vi "Transfer_FLSH_Format.vi"(11 "FLSH Outputs":T1={"t"=0.0, "p"=0.0, "D"=0.0, "Dl"=0.0, "Dv"=0.0, "x"=[0.0, 0.0, 0.0, 0.0, 0.0, 0.0, 0.0, 0.0, 0.0, 0.0, 0.0, 0.0, 0.0, 0.0, 0.0, 0.0, 0.0, 0.0, 0.0, 0.0], "y"=[0.0, 0.0, 0.0, 0.0, 0.0, 0.0, 0.0, 0.0, 0.0, 0.0, 0.0, 0.0, 0.0, 0.0, 0.0, 0.0, 0.0, 0.0, 0.0, 0.0], "q"=0.0, "e"=0.0, "h"=0.0, "s"=0.0, "Cv"=0.0, "Cp"=0.0, "w"=0.0, "ierr"=0, "herr"="", "herr_Length"=0}) -> (3 "Array out":dbl[](array[numeric]))   [LabVIEW 2016]
doc: "Converts output clusters from all FLSH functions to an array of data"
uses:
  Ctl/FLSH_Outputs.ctl
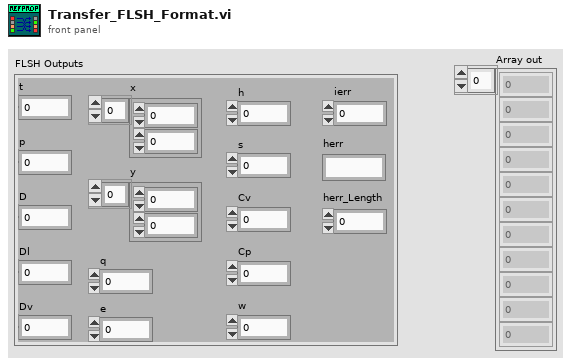
[diagram p1: front panel]
types:
  T1 = typedef "FLSH_Outputs.ctl" = cluster{"t":dbl, "p":dbl, "D":dbl, "Dl":dbl, "Dv":dbl, "x":dbl[], "y":dbl[], "q":dbl, "e":dbl, "h":dbl, "s":dbl, "Cv":dbl, "Cp":dbl, "w":dbl, "ierr":i32, "herr":string, "herr_Length":i32}
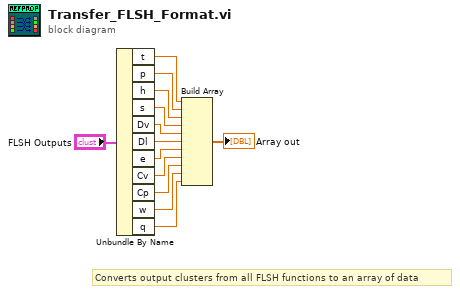
[diagram p0: block diagram]
diagram:
  # "Converts output clusters from all FLSH functions to an array of data"
  n1 = Unbundle By Name("FLSH Outputs") -> ("t"=w11:dbl, "p"=w10:dbl, "h"=w9:dbl, "s"=w8:dbl, "Dv"=w7:dbl, "Dl"=w6:dbl, "e"=w5:dbl, "Cv"=w4:dbl, "Cp"=w3:dbl, "w"=w2:dbl, "q"=w1:dbl)
  n2 = Build Array(w11, w10, w9, w8, w7, w6, w5, w4, w3, w2, w1) -> (→"Array out":dbl[])
